vi "StressDist_circ_calc.vi"(1 "Angle":dbl, 2 "Parameters":dbl[](array[numeric])) -> (0 "Stress":dbl)   [LabVIEW 2016]
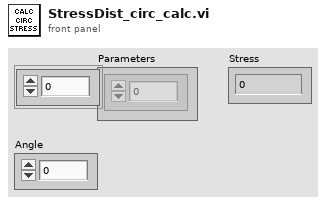
[diagram p1: front panel]
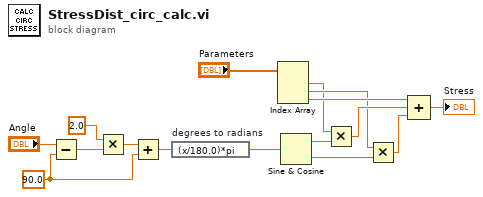
[diagram p0: block diagram]
diagram:
  w1 = 90.0 ("y")
  n1 = Subtract(x="Angle", y=w1) -> (x-y=w4:dbl)
  n2 = Multiply(x=2.0, y=w4) -> (x*y=w3:dbl)
  n3 = Add(x=w3, y=w1) -> (x+y=w2:dbl)
  n4 = expression code="(x/180.0)*pi" "degrees to radians"(w2) -> (w8:dbl)
  n5 = Index Array(array="Parameters") -> (element #1=w10:dbl, element #2=w12:dbl, element #3=w13:dbl)  [unwired: 3 in]
  n6 = Sine & Cosine(0:w8) -> (1:w9:dbl, 2:w11:dbl)
  n7 = Multiply(x=w10, y=w9) -> (x*y=w14:dbl)
  n8 = Multiply(x=w12, y=w11) -> (x*y=w15:dbl)
  n9 = Compound Arithmetic op=ADD(w13, w14, w15) -> (→"Stress":dbl)
